vi "Binary.vi"() -> ()   [LabVIEW 2014]
panel:
  out "String 2":string
  in  "stop":bool
  out "String 3":string
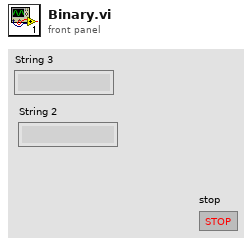
[diagram p1: front panel]
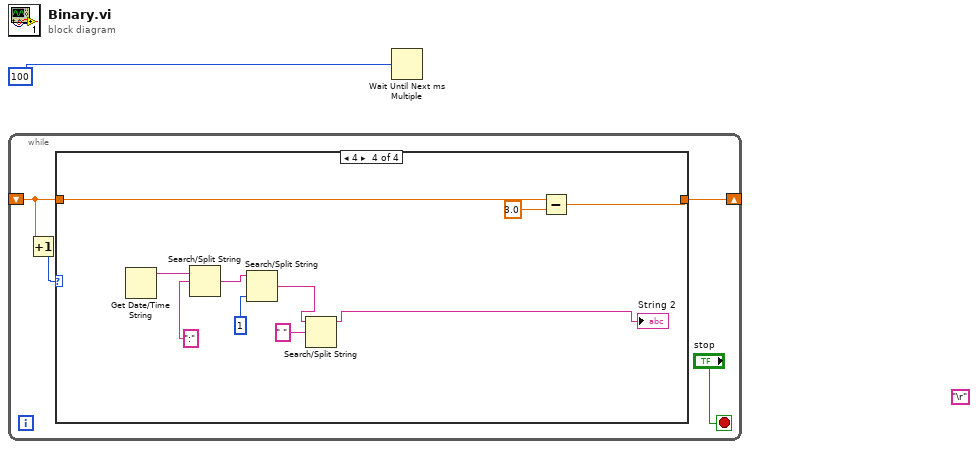
[diagram p0: block diagram]
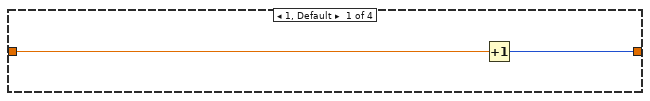
[diagram p2: hidden frame]
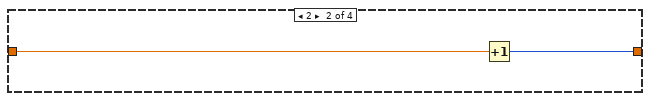
[diagram p3: hidden frame]
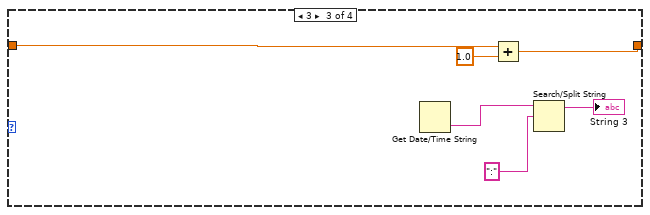
[diagram p4: hidden frame]
diagram:
  (unwired) "\r"
  n1 = while {
    shift-right: [w5] -> _
    shift-left: _ -> [w4]
    stop <- "stop" stop-if-true
    n2 = Increment(x=w4) -> (x+1=w3:u64)
    n3 = case shown="4" w3 {
      tunnel: [w7 w9 w14 w24] -> w5
      tunnel: w4 -> [w6 w8 w15 w25]
      frame 1, Default {
        n4 = Increment(x=w6) -> (x+1=w7:u64)
      }
      frame 2 {
        n5 = Increment(x=w8) -> (x+1=w9:u64)
      }
      frame 3 {
        n6 = Get Date/Time String() -> (time string=w10:string)  [unwired: 3 in, 1 out]
        n7 = Add(x=w15, y=1.0 ("x-y")) -> (x+y=w14:dbl)
        n8 = Search/Split String(string=w10, search string/char (-)=":") -> (substring before match=→"String 3":string)  [unwired: 1 in, 2 out]
      }
      frame 4 {
        n9 = Get Date/Time String() -> (time string=w21:string)  [unwired: 3 in, 1 out]
        n10 = Search/Split String(string=w21, search string/char (-)=":") -> (match + rest of string=w19:string)  [unwired: 1 in, 2 out]
        n11 = Search/Split String(string=w19, offset (0)=1) -> (match + rest of string=w18:string)  [unwired: 1 in, 2 out]
        n12 = Search/Split String(string=w18, search string/char (-)=" ") -> (substring before match=→"String 2":string)  [unwired: 1 in, 2 out]
        n13 = Subtract(x=w25, y=3.0 ("x-y")) -> (x-y=w24:dbl)
      }
    }
  }
  n14 = Wait Until Next ms Multiple(millisecond multiple=100) -> ()  [unwired: 1 out]
